vi "Handle Joystick Case.vi"(1 "Boolean Input":u32[](array[numeric])) -> (0 "Commands":T1=enum."Stop")   [LabVIEW 2018]
uses:
  States.ctl
  Buttons.ctl
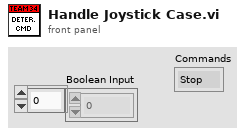
[diagram p1: front panel]
types:
  T1 = typedef "States.ctl" = enum16{"Wait", "Stop", "Limelight Follow", "NavX Reset", "Calibrate Wheels", "Pivot Forward", "Pivot Backward", "Flywheel Forward", "Flywheel Reverse", "FlyDrive Close", "FlyDrive Open", "Pivot Setpoint 0", "Pivot Setpoint 45", "Pivot Setpoint 90"}
  T2 = typedef "Buttons.ctl" = enum16{"A", "B", "X", "Y", "LB", "RB", "Back", "Start", "LS", "RS"}
  T3 = cluster{"Commands":T1, "Buttons":T2[], "Joystick Index":dbl}[]
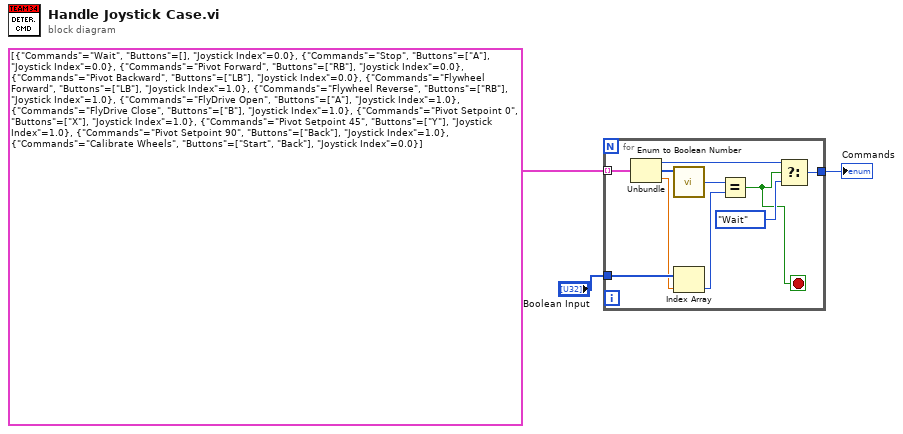
[diagram p0: block diagram]
diagram:
  n1 = for {
    tunnel: "Boolean Input" -> [w13]
    tunnel: [w8] -> w2
    tunnel: T3 [{"Commands"=enum."Wait", "Buttons"=[], "Joystick Index"=0.0}, {"Commands"=enum."Stop", "Buttons"=[enum."A"], "Joystick Index"=0.0}, {"Commands"=enum."Pivot Forward", "Buttons"=[enum."RB"], "Joystick Index"=0.0}, {"Commands"=enum."Pivot Backward", "Buttons"=[enum."LB"], "Joystick Index"=0.0}, {"Commands"=enum."Flywheel Forward", "Buttons"=[enum."LB"], "Joystick Index"=1.0}, {"Commands"=enum."Flywheel Reverse", "Buttons"=[enum."RB"], "Joystick Index"=1.0}, {"Commands"=enum."FlyDrive Open", "Buttons"=[enum."A"], "Joystick Index"=1.0}, {"Commands"=enum."FlyDrive Close", "Buttons"=[enum."B"], "Joystick Index"=1.0}, {"Commands"=enum."Pivot Setpoint 0", "Buttons"=[enum."X"], "Joystick Index"=1.0}, {"Commands"=enum."Pivot Setpoint 45", "Buttons"=[enum."Y"], "Joystick Index"=1.0}, {"Commands"=enum."Pivot Setpoint 90", "Buttons"=[enum."Back"], "Joystick Index"=1.0}, {"Commands"=enum."Calibrate Wheels", "Buttons"=[enum."Start", enum."Back"], "Joystick Index"=0.0}] ("cluster") -> [w7] mode=indexing
    stop <- w4 stop-if-true
    n2 = Unbundle(w7) -> ("Commands"=w10:T1, "Buttons"=w6:T2[], "Joystick Index"=w5:dbl)
    n3 = call "Enum to Boolean Number.vi"("Button Selection"=w6) -> ("number"=w12:u32)  [unwired: 3 in]
    n4 = Index Array(array=w13, index=w5) -> (element=w11:u32)
    n5 = Equal?(x=w12, y=w11) -> (x = y?=w4:bool)
    n6 = Select(t=w10, s=w4, f=States."Wait" ("Commands")) -> (s? t:f=w8:T1)
  }
  "Commands" <- w2
